vi "CalibrationExtract.vi"(11 "Channel":i32) -> (3 "Calibration Values":dbl[](array[numeric]))   [LabVIEW 2012]
uses:
  <vilib>/Utility/file.llb/Read From Spreadsheet File (DBL).vi
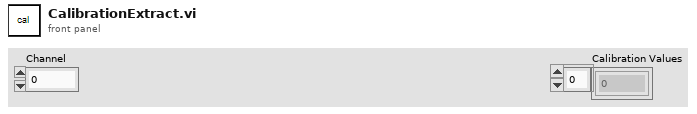
[diagram p1: front panel]
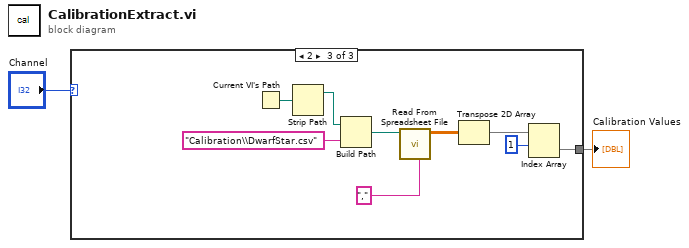
[diagram p0: block diagram]
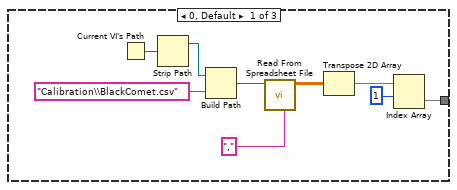
[diagram p2: hidden frame]
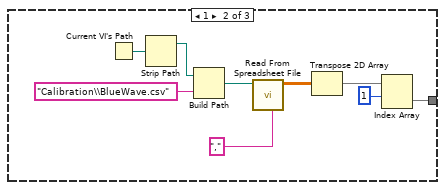
[diagram p3: hidden frame]
diagram:
  n1 = case shown="2" "Channel" {
    tunnel: [w3 w12 w21] -> w1
    frame 0, Default {
      n2 = Current VI's Path() -> (path=w11:path)
      n3 = Strip Path(path=w11) -> (stripped path=w10:path)  [unwired: 1 out]
      n4 = Build Path(base path=w10, name or relative path="Calibration\\BlackComet.csv") -> (appended path=w8:path)
      n5 = call-poly <vilib>:"Read From Spreadsheet File.vi"("delimiter (\\t)"="," ("delimiter (\\t)"), "file path (dialog if empty)"=w8) -> ("all rows"=w6:dbl[][])  [unwired: 5 in, 4 out]
      n6 = Transpose 2D Array(2D array=w6) -> (transposed array=w5:dbl[][])
      n7 = Index Array(array=w5, index (row)=1) -> (element=w3:dbl[])  [unwired: 1 in]
    }
    frame 1 {
      n8 = Current VI's Path() -> (path=w20:path)
      n9 = Strip Path(path=w20) -> (stripped path=w19:path)  [unwired: 1 out]
      n10 = Build Path(base path=w19, name or relative path="Calibration\\BlueWave.csv") -> (appended path=w17:path)
      n11 = call-poly <vilib>:"Read From Spreadsheet File.vi"("delimiter (\\t)"="," ("delimiter (\\t)"), "file path (dialog if empty)"=w17) -> ("all rows"=w15:dbl[][])  [unwired: 5 in, 4 out]
      n12 = Transpose 2D Array(2D array=w15) -> (transposed array=w14:dbl[][])
      n13 = Index Array(array=w14, index (row)=1) -> (element=w12:dbl[])  [unwired: 1 in]
    }
    frame 2 {
      n14 = Current VI's Path() -> (path=w29:path)
      n15 = Strip Path(path=w29) -> (stripped path=w28:path)  [unwired: 1 out]
      n16 = Build Path(base path=w28, name or relative path="Calibration\\DwarfStar.csv") -> (appended path=w26:path)
      n17 = call-poly <vilib>:"Read From Spreadsheet File.vi"("delimiter (\\t)"="," ("delimiter (\\t)"), "file path (dialog if empty)"=w26) -> ("all rows"=w24:dbl[][])  [unwired: 5 in, 4 out]
      n18 = Transpose 2D Array(2D array=w24) -> (transposed array=w23:dbl[][])
      n19 = Index Array(array=w23, index (row)=1) -> (element=w21:dbl[])  [unwired: 1 in]
    }
  }
  "Calibration Values" <- w1
